vi "DAC Configure.vi"(8 "error in":errorcluster, 11 "DAC HeatFlow Temp in":refnum<class "DAC HeatFlow Temp.lvclass">) -> (0 "error out":errorcluster, 3 "DAC HeatFlow Temp out":refnum<class "DAC HeatFlow Temp.lvclass">)   [LabVIEW 2019, in "DAC.lvlib" / "DAC HeatFlow Temp.lvclass"]
uses:
  DAC HeatFlow Temp.lvclass
  C:/Users/krio/Documents/LV_Projects/test-stand/App/DAC/DAC.lvclass
  DAC.lvclass/DAC.ctl
  DAC HeatFlow Temp.lvclass/DAC HeatFlow Temp.ctl
  <vilib>/DAQmx/configure/timing.llb/DAQmx Timing (Sample Clock).vi
  DAC.lvclass
  <vilib>/DAQmx/create/channels.llb/DAQmx Create Channel (AI-Temperature-RTD).vi
  <vilib>/Instr/_visa.llb/VISA Configure Serial Port (Instr).vi
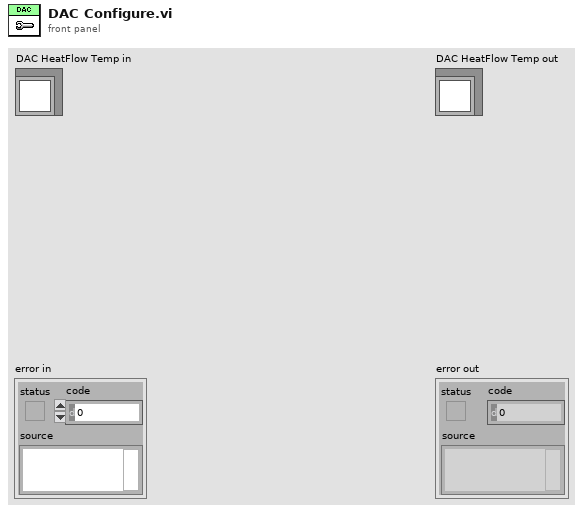
[diagram p1: front panel]
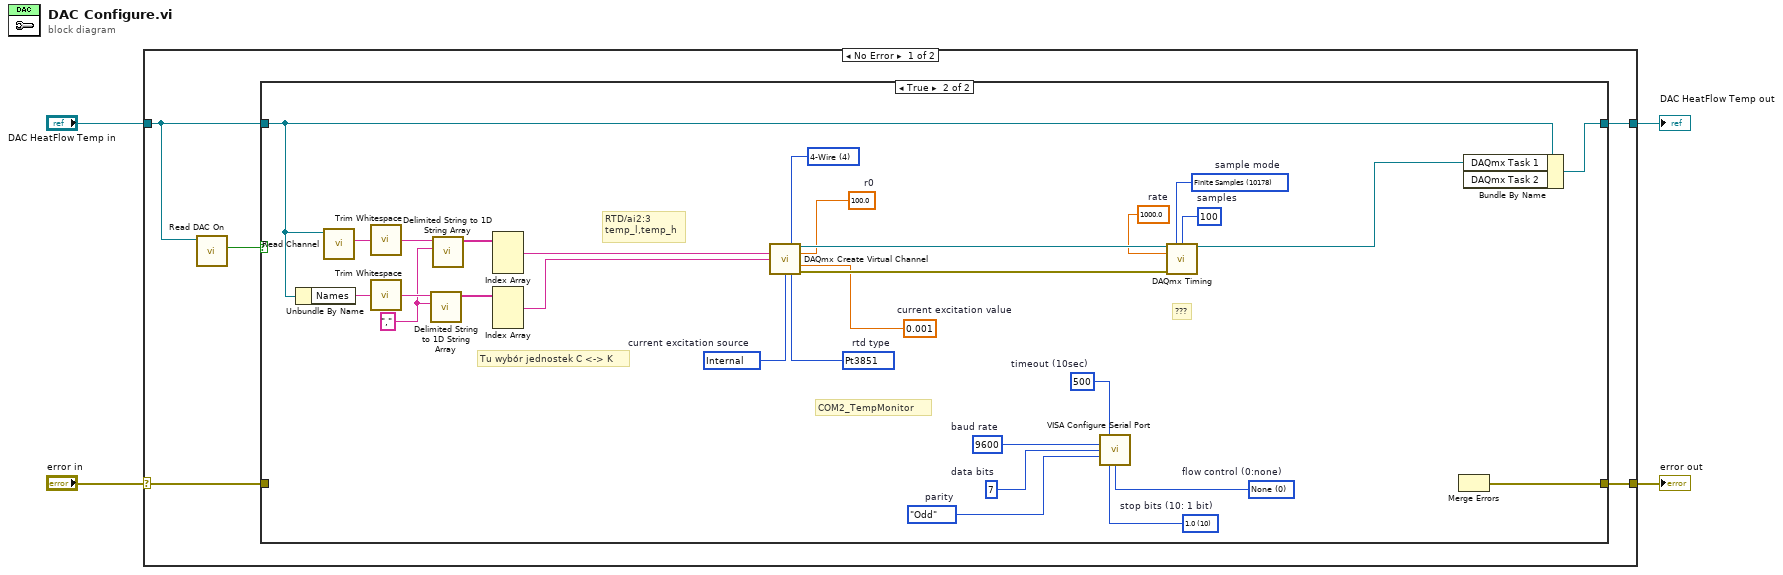
[diagram p0: block diagram]
diagram:
  n1 = case shown="No Error" "error in" {
    selector: "error in" -> [w6 w42]
    tunnel: [w5 w42] -> w4
    tunnel: [w7 w41] -> w3
    tunnel: "DAC HeatFlow Temp in" -> [w9 w41]
    frame No Error {
      n2 = call "Read DAC On.vi"("DAC in"=w9) -> ("DAC On"=w8:bool)  [unwired: 8 in, 2 out]
      n3 = case shown="True" w8 {
        tunnel: w9 -> [w11 w39]
        tunnel: [w11 w40] -> w7
        tunnel: w6 -> [w10 _]
        tunnel: [w10 w23] -> w5
        frame False {
        }
        frame True {
          w12 = u16 0 items=["None", "XON/XOFF", "RTS/CTS", "XON/XOFF & RTS/CTS", "DTR/DSR", "XON/XOFF & DTR/DSR"]  # flow control (0:none)
          w13 = u16 10 items=["1.0"=10, "1.5"=15, "2.0"=20]  # stop bits (10: 1 bit)
          w14 = enum16{"None", "Odd", "Even", "Mark", "Space"}."Odd"  # parity
          w15 = u16 7  # data bits
          w16 = u32 9600  # baud rate
          w17 = u32 500  # timeout (10sec)
          w18 = 0.001  # current excitation value
          w19 = 10071 items=["Pt3750"=12481, "Pt3851"=10071, "Pt3911"=12482, "Pt3916"=10069, "Pt3920"=10053, "Pt3928"=12483, "Custom"=10137]  # rtd type
          w20 = 10200 items=["Internal"=10200, "External"=10167, "None"=10230]  # current excitation source
          w21 = 100.0  # r0
          w22 = 4 items=["2-Wire"=2, "3-Wire"=3, "4-Wire"=4] ("resistance configuration")
          w28 = "," ("delimiter")
          w34 = 100  # samples
          w35 = 1000.0  # rate
          w36 = 10178 items=["Finite Samples"=10178, "Continuous Samples"=10123, "Hardware Timed Single Point"=12522]  # sample mode
          # "COM2_TempMonitor"
          # "Tu wybór jednostek C <-> K"
          # "???"
          # "RTD/ai2:3\ntemp_l,temp_h"
          n4 = Unbundle By Name(w39) -> ("Names"=w31:string)
          n5 = call "Read Channel.vi"("DAC in"=w39) -> ("Channel"=w32:string)  [unwired: 8 in, 2 out]
          n6 = call <vilib>:"Trim Whitespace.vi"("string"=w32) -> ("trimmed string"=w30:string)  [unwired: 1 in]
          n7 = call <vilib>:"Trim Whitespace.vi"("string"=w31) -> ("trimmed string"=w29:string)  [unwired: 1 in]
          n8 = call <vilib>:"Delimited String to 1D String Array.vi"("delimiter"=w28, "delimited string"=w29) -> ("string array"=w26:string[])  [unwired: 9 in]
          n9 = call <vilib>:"Delimited String to 1D String Array.vi"("delimiter"=w28, "delimited string"=w30) -> ("string array"=w27:string[])  [unwired: 9 in]
          n10 = Index Array(array=w27) -> (element #1=w25:string)  [unwired: 3 in, 2 out]
          n11 = Index Array(array=w26) -> (element #1=w24:string)  [unwired: 3 in, 2 out]
          n12 = call-poly <vilib>:"DAQmx Create Virtual Channel.vi"("resistance configuration"=w22, "physical channels"=w25, "r0"=w21, "name to assign"=w24, "current excitation value"=w18, "current excitation source"=w20, "rtd type"=w19) -> ("task out"=w38:refnum<k21>, "error out"=w37:errorcluster)  [unwired: 7 in]
          n13 = call-poly "VISA Configure Serial Port"("timeout (10sec)"=w17, "baud rate (9600)"=w16, "data bits (8)"=w15, "parity (0:none)"=w14, "stop bits (10: 1 bit)"=w13, "flow control (0:none)"=w12) -> ()  [unwired: 8 in, 2 out]
          n14 = call-poly <vilib>:"DAQmx Timing.vi"("task/channels in"=w38, "sample mode"=w36, "samples per channel"=w34, "rate"=w35, "error in"=w37) -> ("task out"=w33:refnum<k21>)  [unwired: 9 in, 1 out]
          n15 = Merge Errors() -> (w23:errorcluster)  [unwired: 2 in]
          n16 = Bundle By Name(cluster=w39, "DAQmx Task 1"=w33) -> (w40:refnum<class "DAC HeatFlow Temp.lvclass">)  [unwired: 1 in]
        }
      }
    }
    frame Error {
    }
  }
  "error out" <- w4
  "DAC HeatFlow Temp out" <- w3
